vi "bmd101Parser_v1.1.vi"() -> ()   [LabVIEW 2016]
doc: "This example performs writes and reads on a serial port, as directed by the user. You can press the Write and Read buttons, and change the Read Count, while the example is running.\n\nThe parameters set for the serial port must match the parameters of the connected instrument or device. In this example, the Read Count parameter specifies the number of bytes that the serial port reads. If there were more bytes at the port than the specified number, those bytes would not be read. If there were less bytes at the port than the specified number, you would receive a timeout error.\n\nThis example expands upon the flow control options for XON and XOFF, allowing the user to choose those control characters. Also, the user can enable or disable a termination character. Some devices require a termination character in order to identify the end of command strings. Some devices send a termination character to signify the end of data to be read. This example shows how you can end the Read operation once a termination character is detected in the buffer and/or append a termination character at the end of the Write data."
uses:
  C:/Program Files/National Instruments/LabVIEW 2016/examples/Instrument IO/Serial/support/Serial - Settings.ctl
  <vilib>/Instr/_visa.llb/VISA Configure Serial Port (Instr).vi
panel:
  out "Stop Loop":bool
  out "Heart Rate":u8[](graph)
  out "Heart Rate":u16[](array[numeric])
  out "Poor Sensor Quality: \nSensor on":bool
  out "Poor Sensor Quality: \nSensor off":bool
  out "ECG":i16[](graph)
  out "return count":u32
  in  "Read Count":u32=960
  in  "Read":bool=TRUE
  in  "Stop":bool
  in  "Serial Settings":T1={"baud rate"=57600, "data bits"=8, "parity"=enum."None", "stop bits"=10, "flow control"=0} {"flow control" items=["None"=0, "XON/XOFF"=1, "RTS/CTS"=2, "DTR/DSR"=4]; "stop bits" items=["1.0"=10, "1.5"=15, "2.0"=20]; "data bits" min=5 max=8 step=1; "baud rate" items=["75"=75, "110"=110, "134"=134, "150"=150, "300"=300, "600"=600, "1200"=1200, "1800"=1800, "2400"=2400, "4800"=4800, "7200"=7200, "9600"=9600, "14400"=14400, "19200"=19200, "28800"=28800, "38400"=38400, "56000"=56000, "57600"=57600, "115200"=115200, "128000"=128000, "230400"=230400]}
  in  "VISA resource name":refnum<visa-resource-name>="bmd101"
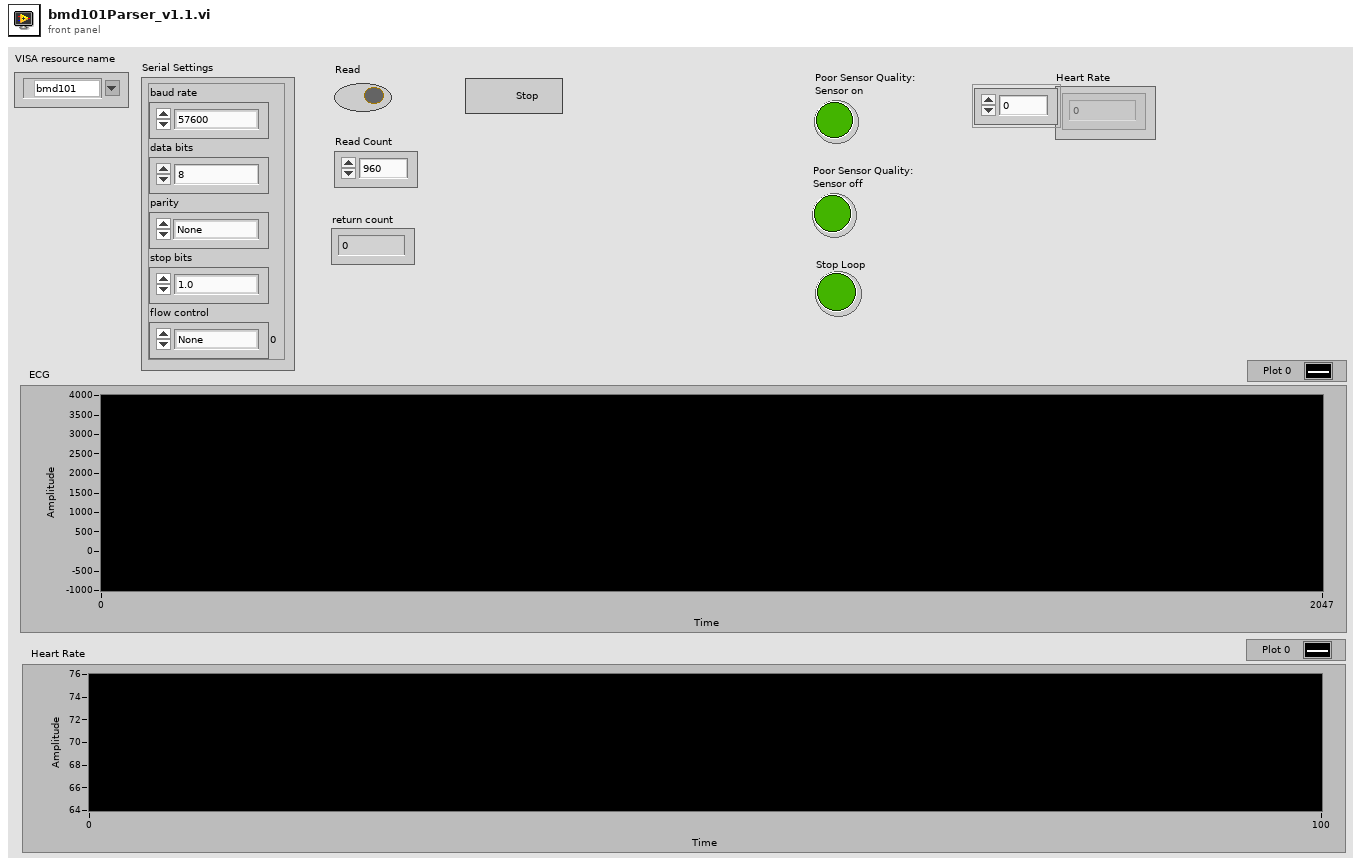
[diagram p1: front panel]
types:
  T1 = typedef "Serial - Settings.ctl" = cluster{"baud rate":u32, "data bits":u16, "parity":enum16{"None", "Odd", "Even", "Mark", "Space"}, "stop bits":u16, "flow control":u16}
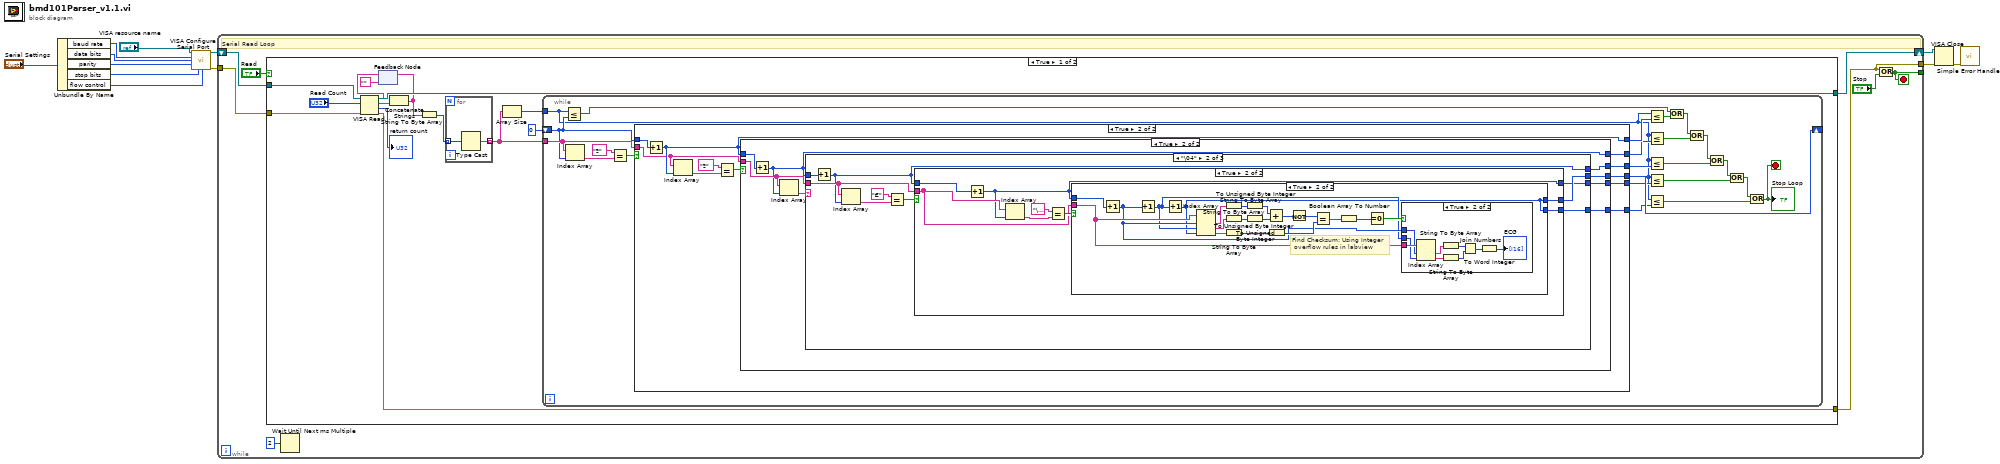
[diagram p0: block diagram]
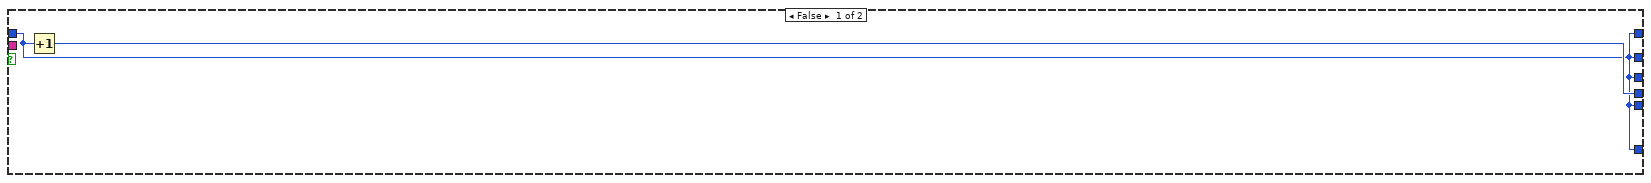
[diagram p2: hidden frame]
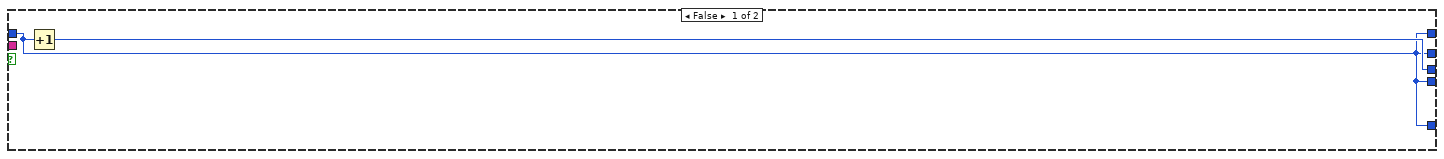
[diagram p3: hidden frame]
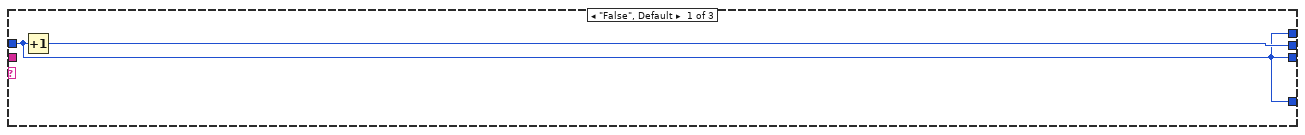
[diagram p4: hidden frame]
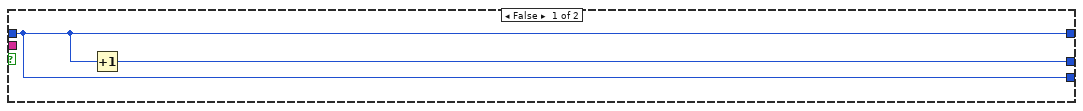
[diagram p5: hidden frame]
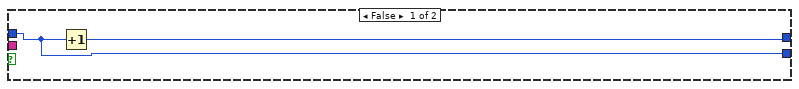
[diagram p6: hidden frame]
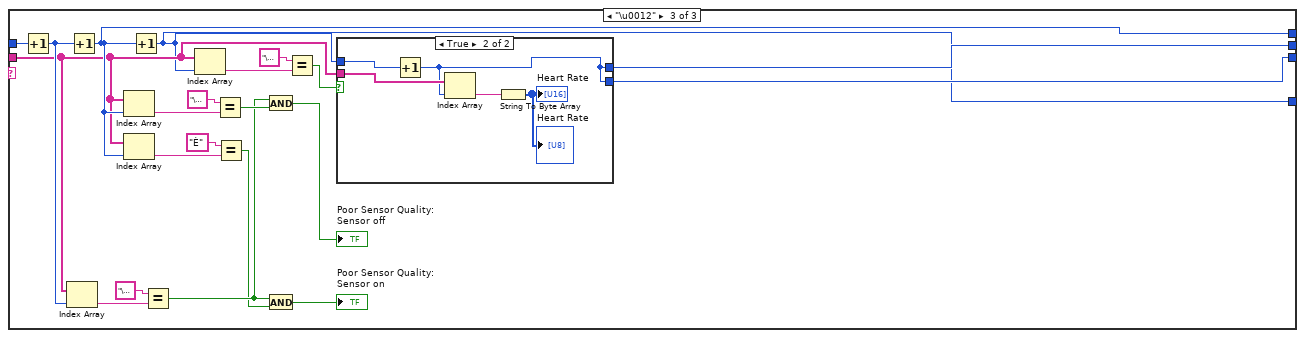
[diagram p8: hidden frame]
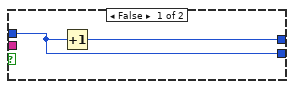
[diagram p9: hidden frame]
diagram:
  n1 = Unbundle By Name("Serial Settings") -> ("baud rate"=w11:u32, "data bits"=w10:u16, "parity"=w9:enum16{"None", "Odd", "Even", "Mark", "Space"}, "stop bits"=w8:u16, "flow control"=w7:u16)
  n2 = call-poly "VISA Configure Serial Port"("VISA resource name"="VISA resource name", "baud rate (9600)"=w11, "data bits (8)"=w10, "parity (0:none)"=w9, "stop bits (10: 1 bit)"=w8, "flow control (0:none)"=w7) -> ("VISA resource name out"=w3:refnum<visa-resource-name>, "error out"=w2:errorcluster)  [unwired: 4 in, 4 out]
  n3 = while {
    shift-right: [w20] -> w4
    shift-left: w3 -> [w16]
    tunnel: w2 -> [w15]
    tunnel: [w18] -> w5
    tunnel: [w14] -> _
    stop <- w14 stop-if-true
    # "Serial Read Loop"
    n4 = case shown="True" "Read" {
      tunnel: [w32 w163] -> w20
      tunnel: w16 -> [w34 w163]
      tunnel: [w30 w162] -> w18
      tunnel: w15 -> [w33 w162]
      frame True {
        n5 = VISA Read(VISA resource name=w34, byte count="Read Count", error in (no error)=w33) -> (VISA resource name out=w32:refnum<visa-resource-name>, read buffer=w29:string, return count=→"return count":u32, error out=w30:errorcluster)
        n6 = feedback #1("") -> (w28:string)
        n7 = Concatenate Strings(w28, w29) -> (w25:string)
        n8 = feedback-in #1(w25) -> ()
        n9 = String To Byte Array(string=w25) -> (unsigned byte array=w26:u8[])
        n10 = for {
          tunnel: w26 -> [w161] mode=indexing
          tunnel: [w160] -> w23 mode=indexing
          n11 = Type Cast(x=w161) -> (*(type *) &x=w160:string)  [unwired: 1 in]
        }
        n12 = Array Size(array=w23) -> (size(s)=w21:i32)
        n13 = while {
          tunnel: w23 -> [w53]
          shift-right: [w57] -> _
          shift-left: 0 -> [w52]
          tunnel: w21 -> [w38]
          stop <- w35 stop-if-true
          n14 = Less Or Equal?(x=w38, y=w52) -> (x <= y?=w50:bool)
          n15 = Index Array(array=w53, index=w52) -> (element=w56:string)
          n16 = Equal?(x="ª", y=w56) -> (x = y?=w54:bool)
          n17 = case shown="True" w54 {
            tunnel: w52 -> [w58 w68]
            tunnel: [w59 w66] -> w57
            tunnel: w53 -> [_ w60]
            tunnel: [w58 w65] -> w51
            tunnel: [w58 w64] -> w48
            tunnel: [w58 w63] -> w45
            tunnel: [w58 w62] -> w42
            tunnel: [w58 w61] -> w39
            frame False {
              n18 = Increment(x=w58) -> (x+1=w59:i32)
            }
            frame True {
              n19 = Increment(x=w68) -> (x+1=w65:i32)
              n20 = Index Array(array=w60, index=w65) -> (element=w70:string)
              n21 = Equal?(x="ª", y=w70) -> (x = y?=w67:bool)
              n22 = case shown="True" w67 {
                tunnel: w65 -> [w71 w74]
                tunnel: [w72 w80] -> w66
                tunnel: w60 -> [_ w79]
                tunnel: [w71 w75] -> w64
                tunnel: [w71 w78] -> w63
                tunnel: [w71 w77] -> w62
                tunnel: [w71 w76] -> w61
                frame False {
                  n23 = Increment(x=w71) -> (x+1=w72:i32)
                }
                frame True {
                  n24 = Increment(x=w74) -> (x+1=w75:i32)
                  n25 = Index Array(array=w79, index=w75) -> (element=w73:string)
                  n26 = case shown="\"\\04\"" w73 {
                    tunnel: w75 -> [w81 w88 w151]
                    tunnel: [w82 w87 w133] -> w80
                    tunnel: w79 -> [_ w86 w135]
                    tunnel: [w81 w85 w137] -> w78
                    tunnel: [w81 w84 w134] -> w77
                    tunnel: [w81 w83 w132] -> w76
                    frame "False", Default {
                      n27 = Increment(x=w81) -> (x+1=w82:i32)
                    }
                    frame "\u0004" {
                      n28 = Increment(x=w88) -> (x+1=w85:i32)
                      n29 = Index Array(array=w86, index=w85) -> (element=w89:string)
                      n30 = Equal?(x="€", y=w89) -> (x = y?=w90:bool)
                      n31 = case shown="True" w90 {
                        tunnel: w85 -> [w92 w98]
                        tunnel: [w93 w97] -> w87
                        tunnel: w86 -> [_ w96]
                        tunnel: [w92 w95] -> w84
                        tunnel: [w92 w94] -> w83
                        frame False {
                          n32 = Increment(x=w92) -> (x+1=w93:i32)
                        }
                        frame True {
                          n33 = Increment(x=w98) -> (x+1=w95:i32)
                          n34 = Index Array(array=w96, index=w95) -> (element=w99:string)
                          n35 = Equal?(x="\u0002", y=w99) -> (x = y?=w100:bool)
                          n36 = case shown="True" w100 {
                            tunnel: w95 -> [w102 w107]
                            tunnel: [w103 w104] -> w97
                            tunnel: w96 -> [_ w108]
                            tunnel: [w102 w104] -> w94
                            frame False {
                              n37 = Increment(x=w102) -> (x+1=w103:i32)
                            }
                            frame True {
                              # "Find Checksum: Using Integer\n overflow rules in labview"
                              n38 = Increment(x=w107) -> (x+1=w106:i32)
                              n39 = Increment(x=w106) -> (x+1=w105:i32)
                              n40 = Increment(x=w105) -> (x+1=w104:i32)
                              n41 = Index Array(array=w108, index #1=w106, index #2=w105, index #3=w104) -> (element #1=w122:string, element #2=w121:string, element #3=w115:string)
                              n42 = String To Byte Array(string=w122) -> (unsigned byte array=w120:u8[])
                              n43 = String To Byte Array(string=w121) -> (unsigned byte array=w119:u8[])
                              n44 = String To Byte Array(string=w115) -> (unsigned byte array=w114:u8[])
                              n45 = To Unsigned Byte Integer(number=w120) -> (unsigned 8bit integer=w118:u8[])
                              n46 = To Unsigned Byte Integer(number=w119) -> (unsigned 8bit integer=w117:u8[])
                              n47 = Add(x=w118, y=w117) -> (x+y=w116:u8[])
                              n48 = To Unsigned Byte Integer(number=w114) -> (unsigned 8bit integer=w112:u8[])
                              n49 = Not(x=w116) -> (.not. x?=w113:u8[])
                              n50 = Equal?(x=w113, y=w112) -> (x = y?=w111:bool[])
                              n51 = Boolean Array To Number(Boolean array=w111) -> (number=w110:u32)
                              n52 = Equal To 0?(x=w110) -> (x = 0?=w109:bool)
                              n53 = case shown="True" w109 {
                                tunnel: w108 -> [_ w131]
                                tunnel: w106 -> [_ w124]
                                tunnel: w105 -> [_ w123]
                                frame False {
                                }
                                frame True {
                                n54 = Index Array(array=w131, index #1=w124, index #2=w123) -> (element #1=w130:string, element #2=w129:string)
                                n55 = String To Byte Array(string=w130) -> (unsigned byte array=w128:u8[])
                                n56 = String To Byte Array(string=w129) -> (unsigned byte array=w127:u8[])
                                n57 = Join Numbers(hi=w128, lo=w127) -> ((hi.lo)=w126:u16[])
                                n58 = To Word Integer(number=w126) -> (16bit integer=→"ECG":i16[])
                                }
                              }
                            }
                          }
                        }
                      }
                    }
                    frame "\u0012" {
                      n59 = Increment(x=w151) -> (x+1=w147:i32)
                      n60 = Index Array(array=w135, index=w147) -> (element=w150:string)
                      n61 = Increment(x=w147) -> (x+1=w137:i32)
                      n62 = Index Array(array=w135, index=w137) -> (element=w148:string)
                      n63 = Index Array(array=w135, index=w137) -> (element=w145:string)
                      n64 = Increment(x=w137) -> (x+1=w132:i32)
                      n65 = Equal?(x="\u0002", y=w150) -> (x = y?=w142:bool)
                      n66 = Index Array(array=w135, index=w132) -> (element=w138:string)
                      n67 = Equal?(x="\u0000", y=w148) -> (x = y?=w144:bool)
                      n68 = Equal?(x="È", y=w145) -> (x = y?=w141:bool)
                      n69 = And(x=w142, y=w144) -> (x .and. y?=→"Poor Sensor Quality: \nSensor off":bool)
                      n70 = And(x=w142, y=w141) -> (x .and. y?=→"Poor Sensor Quality: \nSensor on":bool)
                      n71 = Equal?(x="\u0003", y=w138) -> (x = y?=w136:bool)
                      n72 = case shown="True" w136 {
                        tunnel: w132 -> [w153 w159]
                        tunnel: w135 -> [_ w158]
                        tunnel: [w153 w157] -> w134
                        tunnel: [w154 w157] -> w133
                        frame False {
                          n73 = Increment(x=w153) -> (x+1=w154:i32)
                        }
                        frame True {
                          n74 = Increment(x=w159) -> (x+1=w157:i32)
                          n75 = Index Array(array=w158, index=w157) -> (element=w156:string)
                          n76 = String To Byte Array(string=w156) -> (unsigned byte array=→"Heart Rate" →"Heart Rate":u8[])
                        }
                      }
                    }
                  }
                }
              }
            }
          }
          n77 = Less Or Equal?(x=w38, y=w51) -> (x <= y?=w49:bool)
          n78 = Less Or Equal?(x=w38, y=w48) -> (x <= y?=w46:bool)
          n79 = Less Or Equal?(x=w38, y=w45) -> (x <= y?=w43:bool)
          n80 = Less Or Equal?(x=w38, y=w42) -> (x <= y?=w40:bool)
          n81 = Less Or Equal?(x=w38, y=w39) -> (x <= y?=w36:bool)
          n82 = Or(x=w50, y=w49) -> (x .or. y?=w47:bool)
          n83 = Or(x=w47, y=w46) -> (x .or. y?=w44:bool)
          n84 = Or(x=w44, y=w43) -> (x .or. y?=w41:bool)
          n85 = Or(x=w41, y=w40) -> (x .or. y?=w37:bool)
          n86 = Or(x=w37, y=w36) -> (x .or. y?=w35:bool)
          "Stop Loop" <- w35
        }
      }
      frame False {
      }
    }
    n87 = Wait Until Next ms Multiple(millisecond multiple=u32 2 ("milliseconds to wait")) -> ()  [unwired: 1 out]
    n88 = Or(x=w18, y="Stop") -> (x .or. y?=w14:bool)
  }
  n89 = VISA Close(VISA resource name=w4, error in (no error)=w5) -> (error out=w1:errorcluster)
  n90 = call <vilib>:"Simple Error Handler.vi"("error in (no error)"=w1) -> ()  [unwired: 1 in, 8 out]
